vi "Data Count.vi"(8 "error in (no error)":errorcluster, 10 "Data Count":i32, 11 "Test Caller in":refnum<class "Test Caller.lvclass">) -> (0 "error out":errorcluster, 3 "Test Caller out":refnum<class "Test Caller.lvclass">)   [LabVIEW 2022 SP3, in "Scratchpad.lvlib" / "Test Caller.lvlib" / "Test Caller.lvclass"]
uses:
  Test Caller.lvclass
  Test Caller.lvclass/Test Caller.ctl
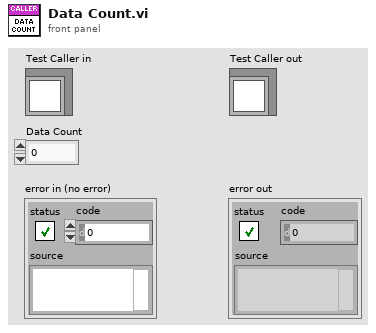
[diagram p1: front panel]
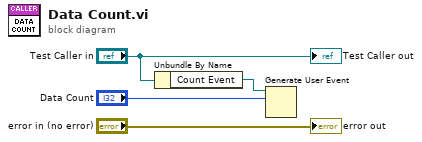
[diagram p0: block diagram]
diagram:
  n1 = Unbundle By Name("Test Caller in") -> ("Count Event"=w2:refnum<user-event>)
  n2 = Generate User Event(user event=w2, event data cluster="Data Count") -> ()  [unwired: 2 in, 2 out]
  "error out" <- "error in (no error)"
  "Test Caller out" <- "Test Caller in"
